vi "DriveModuleReadEncoder.vi"(8 "error in":errorcluster, 11 "ModualNamePrefix":i32) -> (0 "error out":errorcluster, 2 "SWERVE_DRIVE_MODULE_POSITION":T1={"Distance"=0.0, "Angle"={"VALUE"=0.0, "COS"=1.0, "SIN"=0.0}, "P"=FALSE} {"Angle"."SIN" format="%13.4f"; "Angle"."COS" format="%13.4f"; "Angle"."VALUE" format="%13.4f"}, 3 "SWERVE_DRIVE_MODULE_STATE":T3={"Speed"=0.0, "Angle"={"VALUE"=0.0, "COS"=1.0, "SIN"=0.0}} {"Angle"."SIN" format="%13.4f"; "Angle"."COS" format="%13.4f"; "Angle"."VALUE" format="%13.4f"})   [LabVIEW 2023]
uses:
  <vilib>/Rock Robotics/WPI/ThirdParty/JAS_Junk/TrajLib/TypeDef/SWERVE_DRIVE_MODULE_STATE.ctl
  <vilib>/Rock Robotics/WPI/ThirdParty/JAS_Junk/TrajLib/TypeDef/ROTATION2D.ctl
  <vilib>/Rock Robotics/WPI/ThirdParty/JAS_Junk/TrajLib/TypeDef/SWERVE_DRIVE_MODULE_POSITION.ctl
  <vilib>/Rock Robotics/WPI/ThirdParty/JAS_Junk/TrajLib/Conv_Deg_Radians.vi
  <vilib>/Rock Robotics/WPI/ThirdParty/JAS_Junk/TrajLib/Rotation2d_CreateAngle.vi
  DriveGlobal.vi
  <vilib>/Rock Robotics/WPI/ThirdParty/Phoenix6/Phoenix6_Device_RefNumRegistryGet.vi
  <vilib>/Rock Robotics/WPI/MotorControl/WPI_MotorControlRefNum Registry Get.vi
  <vilib>/Rock Robotics/WPI/ThirdParty/Phoenix6/getters/GetCANcoder_AbsPosition.vi
  <vilib>/Rock Robotics/Network Tables/NT Write Number.vi
  <vilib>/Rock Robotics/WPI/ThirdParty/REV Robotics/REVLib/SubVI/Public/SPARK Get Encoder Status Position.vi
  <vilib>/Rock Robotics/WPI/ThirdParty/REV Robotics/REVLib/SubVI/Public/SPARK Get Encoder Status Velocity.vi
  <vilib>/Rock Robotics/WPI/ThirdParty/JAS_Junk/TrajLib/Trajectory_Library.lvlib
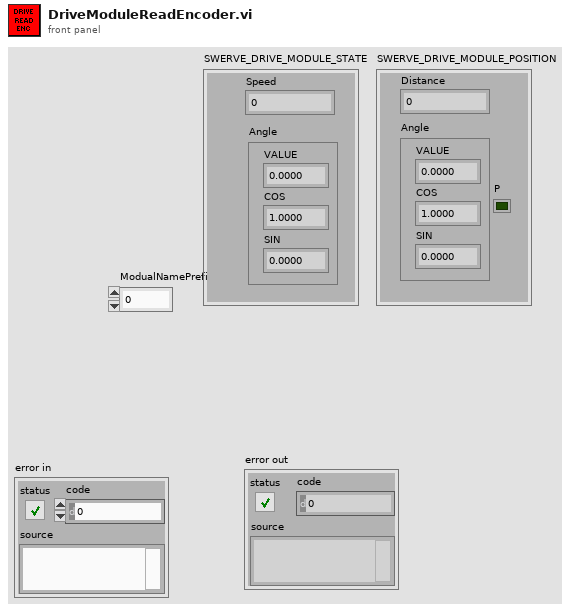
[diagram p1: front panel]
types:
  T1 = typedef "Trajectory_Library.lvlib/SWERVE_DRIVE_MODULE_POSITION.ctl" = cluster{"Distance":dbl, "Angle":T2, "P":bool}
  T2 = typedef "Trajectory_Library.lvlib/ROTATION2D.ctl" = cluster{"VALUE":dbl, "COS":dbl, "SIN":dbl}
  T3 = typedef "Trajectory_Library.lvlib/SWERVE_DRIVE_MODULE_STATE.ctl" = cluster{"Speed":dbl, "Angle":T2}
  T4 = typedef "WPI_MotorControlDeviceRef.ctl" = cluster{"DeviceStatus":errorcluster, "Type":T5, "PWM":cluster{"PWM Channel":T6, "DeadBand":T7}, "CAN":cluster{"Device Number":u8, "SetOutput VI Ref":variant, "GetOutput VI Ref":variant, "Enable VI Ref":variant, "Disable VI Ref":variant, "Data":variant}, "Invert":bool, "DIO PWM":cluster{"PWM \"Enable\" Channel":T6, "DIOChannel":T8, "PWM Rate":dbl}}
  T5 = typedef "WPI_MotorControlType.ctl" = enum16{"PWM", "CAN", "DIO PWM"}
  T6 = typedef "FPGA_DIOPWMChannel.ctl" = enum8{"PWM 0", "PWM 1", "PWM 2", "PWM 3", "PWM 4", "PWM 5", "PWM 6", "PWM 7", "PWM 8", "PWM 9", "PWM MXP 0", "PWM MXP 1", "PWM MXP 2", "PWM MXP 3", "PWM MXP 4", "PWM MXP 5", "PWM MXP 6", "PWM MXP 7", "PWM MXP 8", "PWM MXP 9", "Invalid"}
  T7 = typedef "WPI_PWMDeadband.ctl" = cluster{"Name":string, "maxPositivePwm":i32, "minPositivePwm":i32, "centerPwm":i32, "maxNegativePwm":i32, "minNegativePwm":i32, "angularRange":u16}
  T8 = typedef "FPGA_DIOChannel.ctl" = enum8{"DIO 0", "DIO 1", "DIO 2", "DIO 3", "DIO 4", "DIO 5", "DIO 6", "DIO 7", "DIO 8", "DIO 9", "DIO MXP 0", "DIO MXP 1", "DIO MXP 2", "DIO MXP 3", "DIO MXP 4", "DIO MXP 5", "DIO MXP 6", "DIO MXP 7", "DIO MXP 8", "DIO MXP 9", "DIO MXP 10", "DIO MXP 11", "DIO MXP 12", "DIO MXP 13", "DIO MXP 14", "DIO MXP 15", "SPI Port CS1", "SPI Port CS2", "SPI Port CS3", "SPI Port MISO", "SPI Port MOSI", "Invalid"}
  T9 = typedef "DeviceReference.ctl" = cluster{"CANbus Name":string, "Device Encoding":u32, "Device Name":string}
  T10 = cluster{"Value":dbl, "System Timestamp":dbl, "CANivore Timestamp":dbl, "ECU Timestamp":dbl}
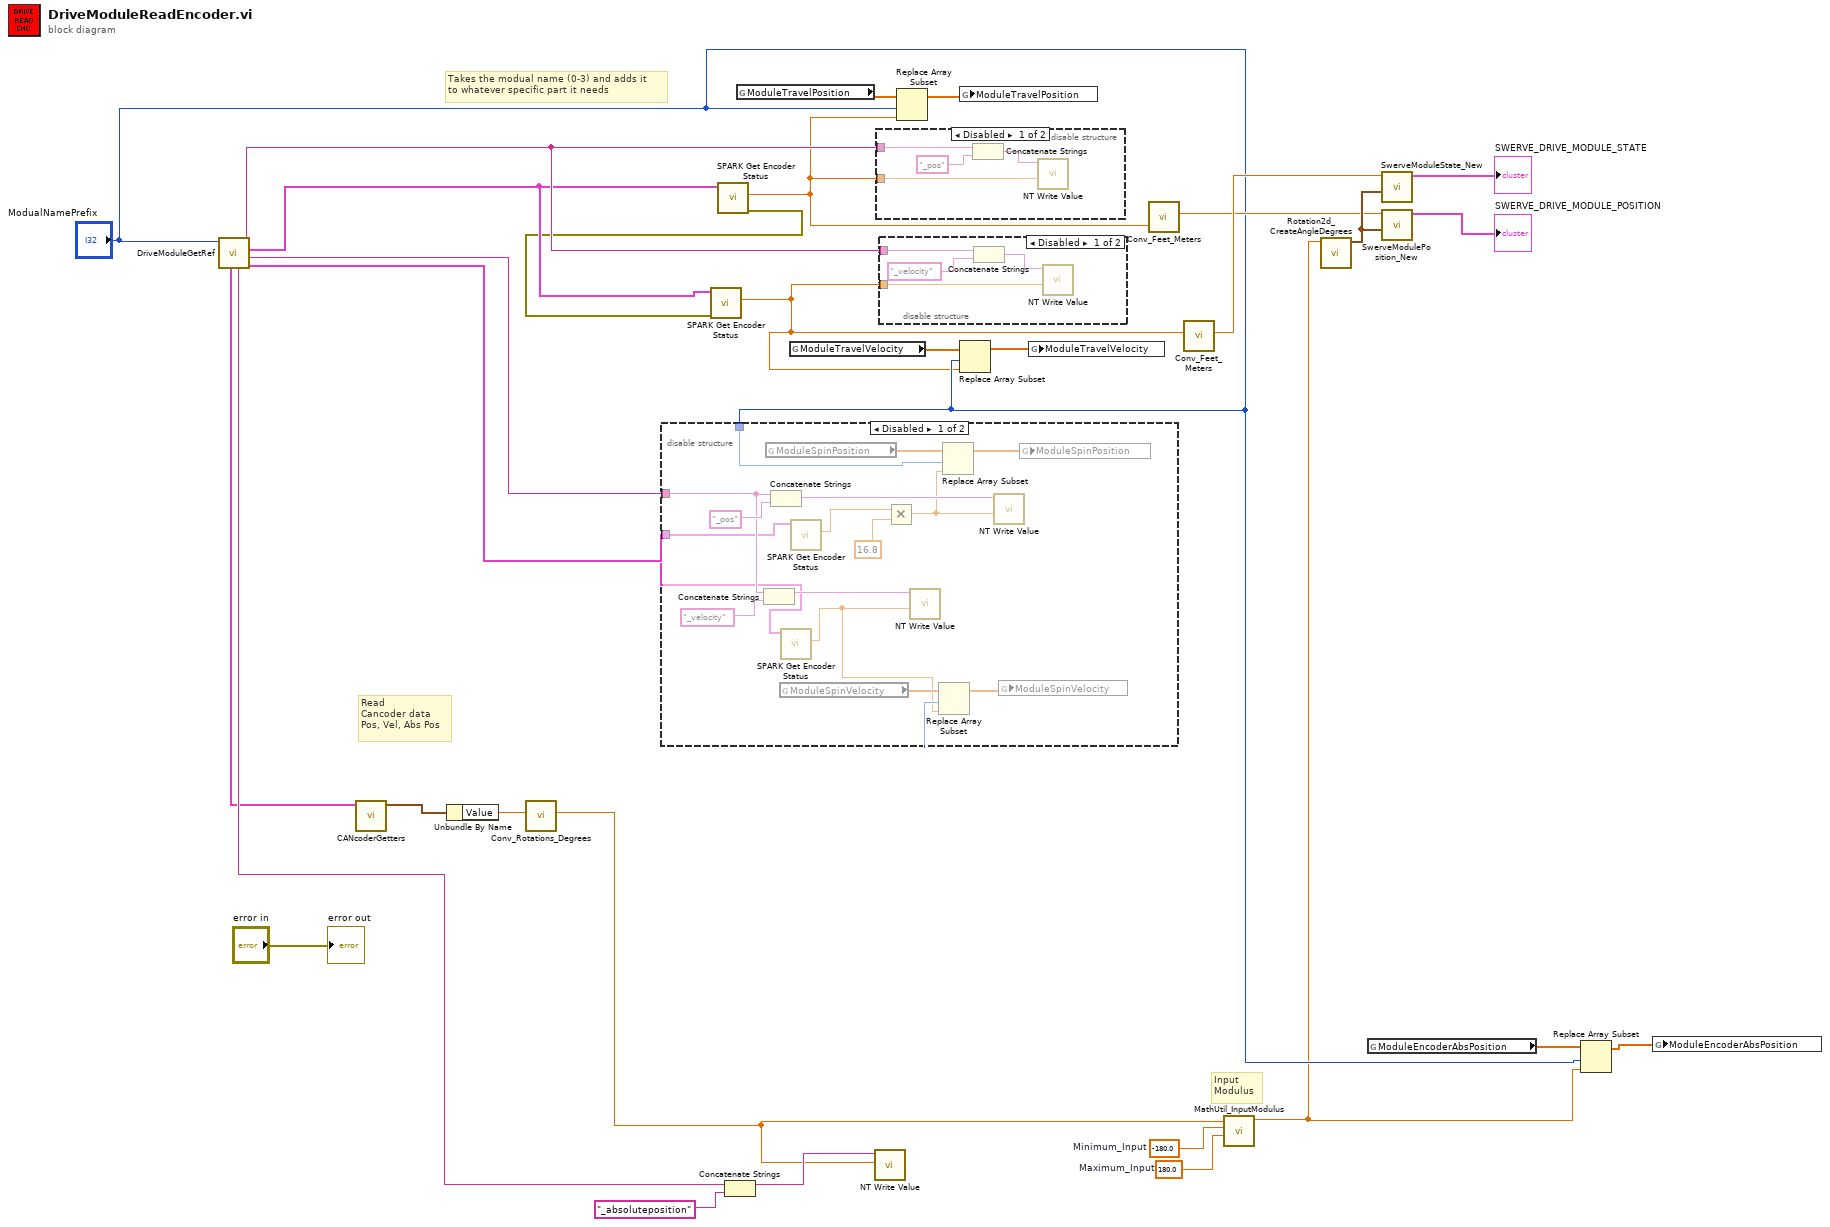
[diagram p0: block diagram]
diagram:
  w24 = -180.0  # Minimum_Input
  w23 = 180.0  # Maximum_Input
  # "Read\nCancoder data\nPos, Vel, Abs Pos"
  # "Input\nModulus"
  # "Takes the modual name (0-3) and adds it \nto whatever specific part it needs"
  n1 = call "DriveModuleGetRef.vi"("ModualNamePrefix"="ModualNamePrefix") -> ("SpinMot"=w16:T4, "SpinStr"=w18:string, "TravMot"=w7:T4, "TravStr"=w17:string, "EncStr"=w15:string, "SpinAbsAngle"=w4:T9)  [unwired: 5 in]
  n2 = call-poly <vilib>:"CANcoderGetters.vi"("DeviceReference"=w4) -> ("Output"=w3:T10)  [unwired: 9 in, 1 out]
  n3 = Unbundle By Name(w3) -> ("Value"=w2:dbl)
  n4 = call <vilib>:"Conv_Rotations_Degrees.vi"("Rotations"=w2) -> ("Degrees"=w1:dbl)  [unwired: 10 in]
  n5 = disable-structure shown="Disabled" {
    disable-tunnel: w18 -> [w40 _]
    disable-tunnel: w16 -> [w32 _]
    disable-tunnel: "ModualNamePrefix" -> [w34 _]
    frame Disabled {
      n6 = Concatenate Strings(w40, "_velocity" ("refnum name")) -> (w42:string)
      n7 = global read "DriveGlobal.vi" "ModuleSpinPosition"() -> (w39:dbl[])
      n8 = Concatenate Strings(w40, "_pos" ("refnum name")) -> (w44:string)
      n9 = global read "DriveGlobal.vi" "ModuleSpinVelocity"() -> (w36:dbl[])
      n10 = call-poly <vilib>:"SPARK Get Encoder Status.vi"("MotorControlDevRef in"=w32) -> ("Sensor Velocity"=w31:dbl)  [unwired: 7 in, 3 out]
      n11 = call-poly <vilib>:"SPARK Get Encoder Status.vi"("MotorControlDevRef in"=w32) -> ("Sensor Position"=w33:dbl)  [unwired: 7 in, 3 out]
      n12 = Multiply(x=w33, y=16.8) -> (x*y=w37:dbl)
      n13 = call-poly <vilib>:"NT Write Value.vi"("value"=w31, "name"=w42) -> ()  [unwired: 9 in, 1 out]
      n14 = Replace Array Subset(array=w36, new element=w31, index=w34) -> (w35:dbl[])
      n15 = Replace Array Subset(array=w39, new element=w37, index=w34) -> (w38:dbl[])
      n16 = call-poly <vilib>:"NT Write Value.vi"("value"=w37, "name"=w44) -> ()  [unwired: 9 in, 1 out]
      n17 = global write "DriveGlobal.vi" "ModuleSpinVelocity"(w35) -> ()
      n18 = global write "DriveGlobal.vi" "ModuleSpinPosition"(w38) -> ()
    }
    frame Enabled {
    }
  }
  n19 = call-poly <vilib>:"SPARK Get Encoder Status.vi"("MotorControlDevRef in"=w7) -> ("error out"=w5:errorcluster, "Sensor Position"=w8:dbl)  [unwired: 7 in, 2 out]
  n20 = call-poly <vilib>:"SPARK Get Encoder Status.vi"("error in (no error)"=w5, "MotorControlDevRef in"=w7) -> ("Sensor Velocity"=w6:dbl)  [unwired: 6 in, 3 out]
  n21 = Concatenate Strings(w15, "_absoluteposition" ("refnum name")) -> (w28:string)
  n22 = global read "DriveGlobal.vi" "ModuleTravelPosition"() -> (w20:dbl[])
  n23 = global read "DriveGlobal.vi" "ModuleTravelVelocity"() -> (w14:dbl[])
  n24 = call-poly <vilib>:"NT Write Value.vi"("value"=w1, "name"=w28) -> ()  [unwired: 9 in, 1 out]
  n25 = disable-structure shown="Disabled" {
    disable-tunnel: w17 -> [w47 _]
    disable-tunnel: w8 -> [w46 _]
    frame Disabled {
      n26 = Concatenate Strings(w47, "_pos" ("refnum name")) -> (w48:string)
      n27 = call-poly <vilib>:"NT Write Value.vi"("value"=w46, "name"=w48) -> ()  [unwired: 9 in, 1 out]
    }
    frame Enabled {
    }
  }
  n28 = disable-structure shown="Disabled" {
    disable-tunnel: w17 -> [w51 _]
    disable-tunnel: w6 -> [w50 _]
    frame Disabled {
      n29 = Concatenate Strings(w51, "_velocity" ("refnum name")) -> (w52:string)
      n30 = call-poly <vilib>:"NT Write Value.vi"("value"=w50, "name"=w52) -> ()  [unwired: 9 in, 1 out]
    }
    frame Enabled {
    }
  }
  n31 = Replace Array Subset(array=w20, new element=w8, index="ModualNamePrefix") -> (w19:dbl[])
  n32 = global write "DriveGlobal.vi" "ModuleTravelPosition"(w19) -> ()
  n33 = Replace Array Subset(array=w14, new element=w6, index="ModualNamePrefix") -> (w13:dbl[])
  n34 = global write "DriveGlobal.vi" "ModuleTravelVelocity"(w13) -> ()
  n35 = call <vilib>:"Conv_Feet_Meters.vi"("Feet"=w8) -> ("Meters"=w21:dbl)  [unwired: 10 in]
  n36 = call <vilib>:"Conv_Feet_Meters.vi"("Feet"=w6) -> ("Meters"=w22:dbl)  [unwired: 10 in]
  n37 = call <vilib>:"MathUtil_InputModulus.vi"("Maximum_Input"=w23, "Minimum_Input"=w24, "Input"=w1) -> ("modulus"=w9:dbl)  [unwired: 8 in]
  n38 = call <vilib>:"Rotation2d_CreateAngleDegrees.vi"("Angle_Degrees"=w9) -> ("ROTATION"=w27:T2)  [unwired: 10 in]
  n39 = global read "DriveGlobal.vi" "ModuleEncoderAbsPosition"() -> (w12:dbl[])
  n40 = call <vilib>:"SwerveModuleState_New.vi"("ROTATION"=w27, "Speed"=w22) -> ("SWERVE_DRIVE_MODULE_STATE"=→"SWERVE_DRIVE_MODULE_STATE":T3)  [unwired: 9 in]
  n41 = call <vilib>:"SwerveModulePosition_New.vi"("ROTATION"=w27, "Distance"=w21) -> ("SWERVE_DRIVE_MODULE_POSITION"=→"SWERVE_DRIVE_MODULE_POSITION":T1)  [unwired: 9 in]
  n42 = Replace Array Subset(array=w12, new element=w9, index="ModualNamePrefix") -> (w11:dbl[])
  n43 = global write "DriveGlobal.vi" "ModuleEncoderAbsPosition"(w11) -> ()
  "error out" <- "error in"
